vi "TestODP.vi"() -> ()   [LabVIEW 2018]
uses:
  State.ctl
  Constraints.ctl
  TrapezoidalProfile.lvclass
panel:
  out "Waveform Graph":cluster{dbl, dbl, dbl[][]}(graph)
  out "Array":dbl[][](array[numeric])
  in  "Constraints":T1
  in  "Unprofiled Goal":T2
  in  "Initial":T2
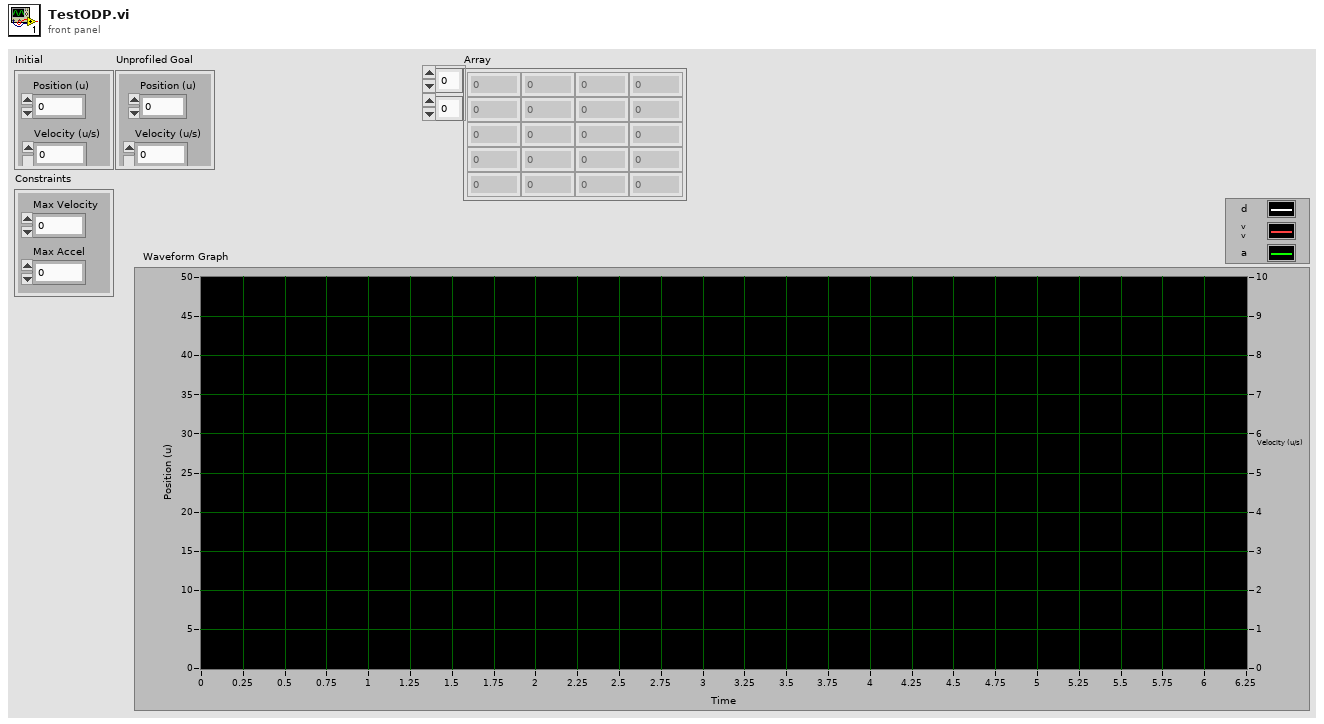
[diagram p1: front panel]
types:
  T1 = typedef "TrapezoidalProfile.lvclass/Constraints.ctl" = cluster{"Max Velocity":dbl, "Max Accel":dbl}
  T2 = typedef "TrapezoidalProfile.lvclass/State.ctl" = cluster{"Position (u)":dbl, "Velocity (u/s)":dbl}
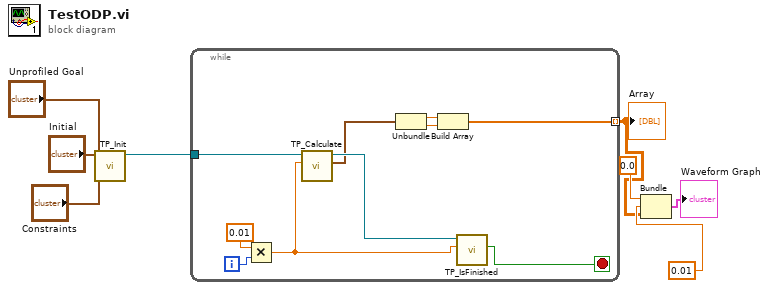
[diagram p0: block diagram]
diagram:
  n1 = call "TP_Init.vi"("Constraints"="Constraints", "Unprofiled Goal"="Unprofiled Goal", "Initial"="Initial") -> ("TrapezoidalProfile out"=w5:refnum<class "TrapezoidalProfile.lvclass">)  [unwired: 7 in, 1 out]
  n2 = while {
    tunnel: w5 -> [w18]
    tunnel: [w15] -> w2 mode=indexing
    i -> [w17]
    stop <- w14 stop-if-true
    n3 = Multiply(x=0.01, y=w17) -> (x*y=w12:dbl)
    n4 = call "TP_Calculate.vi"("t"=w12, "TrapezoidalProfile in"=w18) -> ("Output"=w10:T2, "TrapezoidalProfile out"=w13:refnum<class "TrapezoidalProfile.lvclass">)  [unwired: 7 in, 1 out]
    n5 = Unbundle(w10) -> ("Position (u)"=w16:dbl, "Velocity (u/s)"=w9:dbl)
    n6 = Build Array(w16, w9) -> (w15:dbl[])
    n7 = call "TP_IsFinished.vi"("t"=w12, "TrapezoidalProfile in"=w13) -> ("Is Finished?"=w14:bool)  [unwired: 7 in, 2 out]
  }
  "Array" <- w2
  n8 = Bundle(0.0, 0.01, w2) -> (→"Waveform Graph":cluster{dbl, dbl, dbl[][]})  [unwired: 1 in]
